vi "Label Targets2.vi"(6 "Edges":cluster{"X":sgl, "Y":sgl}[](array[cluster]), 8 "Line":T1, 9 "Annotate":bool, 10 "Results":T3 {"Score" format="%#_3g"; "Pixels"."Rectangle"."Numeric 5" format="%#_3g"; "Pixels"."Rectangle"."Numeric 3" format="%#_3g"; "Pixels"."Rectangle"."Numeric 2" format="%#_3g"; "Pixels"."Rectangle"."Numeric" format="%#_3g"; "Normalized"."Rectangle"."Numeric 5" format="%#_2g"; "Normalized"."Rectangle"."Numeric 3" format="%#_2g"; "Normalized"."Rectangle"."Numeric 2" format="%#_2g"; "Normalized"."Rectangle"."Numeric" format="%#_2g"; "Normalized"."Center"."?" format="%#_3g"; "Normalized"."Center"."?" format="%#_3g"; "Distance (ft)" format="%#_3g"}, 11 "Image in":T2) -> (3 "Image out":T2)   [LabVIEW 2016]
doc: "Draw text values near or on the particle and draws a square around the target stripes.."
uses:
  <vilib>/vision/Image Controls.llb/IMAQ Image.ctl
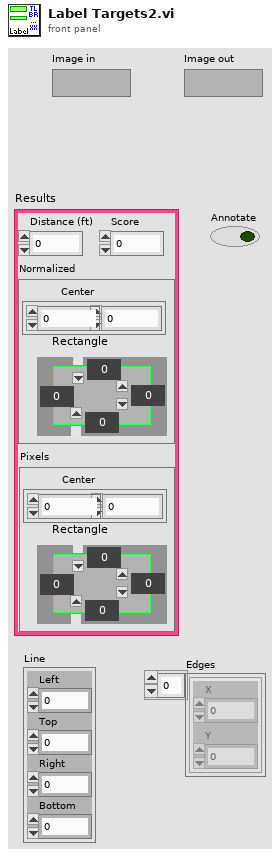
[diagram p1: front panel]
types:
  T1 = cluster{"Left":dbl, "Top":dbl, "Right":dbl, "Bottom":dbl}
  T2 = typedef "IMAQ Image.ctl" = refnum<image>
  T3 = cluster{"Distance (ft)":dbl, "Score":dbl, "Normalized":cluster{"Center":cluster{dbl, dbl}, "Rectangle":cluster{"Numeric":dbl, "Numeric 2":dbl, "Numeric 3":dbl, "Numeric 5":dbl}}, "Pixels":cluster{"Center":cluster{dbl, dbl}, "Rectangle":cluster{"Numeric":dbl, "Numeric 2":dbl, "Numeric 3":dbl, "Numeric 5":dbl}}}
  T4 = cluster{"Desired Font (Application)":enum16{"User-specified Font", "Application Font", "System Font", "Dialog Font"}, "[User-specified Font]":cluster{"Font Name":string, "Size":i16, "Strikeout?":bool, "Italic?":bool, "Underline?":bool, "Outline?":bool, "Shadow?":bool, "Bold?":bool, "Rotation Angle":dbl}, "Horizontal Alignment":i16, "Vertical Alignment":i16}
  T5 = cluster{"Center":cluster{dbl, dbl}, "Rectangle":cluster{"Numeric":dbl, "Numeric 2":dbl, "Numeric 3":dbl, "Numeric 5":dbl}}
  T6 = cluster{"Numeric":dbl, "Numeric 2":dbl, "Numeric 3":dbl, "Numeric 5":dbl}
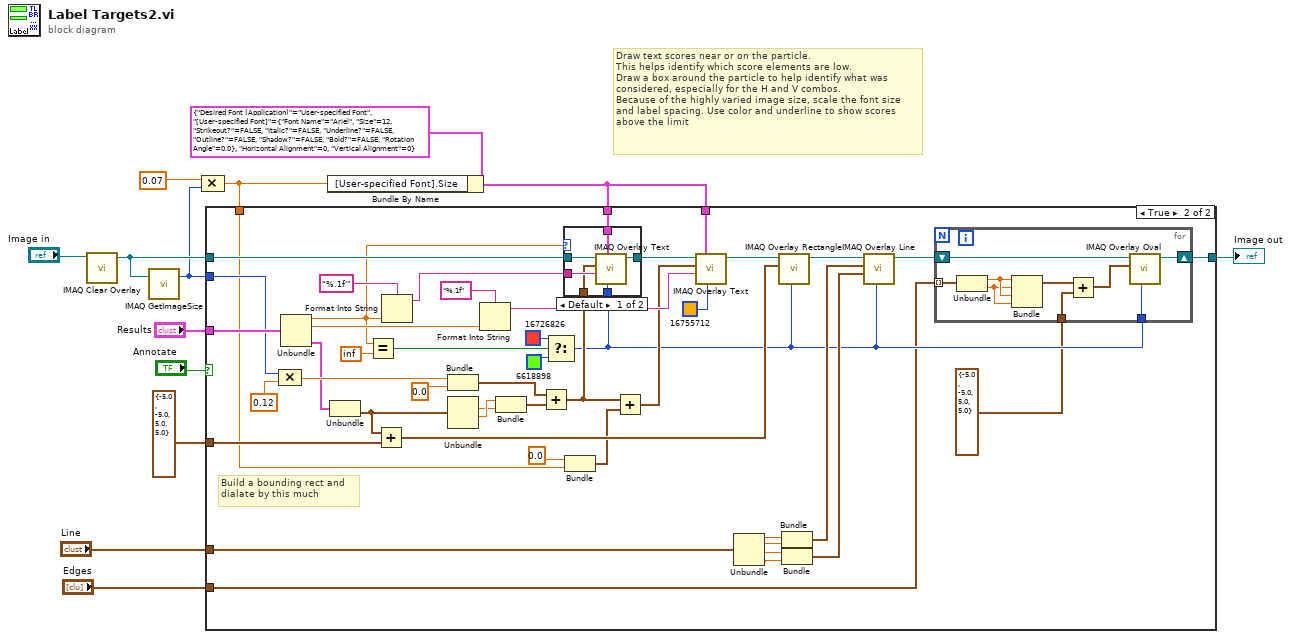
[diagram p0: block diagram]
diagram:
  # "Draw text scores near or on the particle.\nThis helps identify which score elements are low.\nDraw a box around the particle to help identify what was\nconsidered, especially for the H and V combos.\nBecause of the highly varied image size, scale the font size\nand label spacing. Use color and underline to show scores\nabove the limit"
  n1 = call "IMAQ Clear Overlay"("Image"="Image in") -> ("Image Out"=w8:T2)  [unwired: 2 in, 8 out]
  n2 = call "IMAQ GetImageSize"("Image"=w8) -> ("Y Resolution"=w7:i32)  [unwired: 3 in, 2 out]
  n3 = Compound Arithmetic op=MULTIPLY(0.07, w7) -> (w3:dbl)
  n4 = Bundle By Name(cluster=T4 {"Desired Font (Application)"=enum."User-specified Font", "[User-specified Font]"={"Font Name"="Ariel", "Size"=12, "Strikeout?"=FALSE, "Italic?"=FALSE, "Underline?"=FALSE, "Outline?"=FALSE, "Shadow?"=FALSE, "Bold?"=FALSE, "Rotation Angle"=0.0}, "Horizontal Alignment"=0, "Vertical Alignment"=0} ("Font, Size & Style"), "[User-specified Font].Size"=w3) -> (w4:T4)
  n5 = case shown="True" "Annotate" {
    tunnel: [w14 w19] -> w13
    tunnel: "Results" -> [_ w61]
    tunnel: w8 -> [w14 w60]
    tunnel: w4 -> [_ w49]
    tunnel: w7 -> [_ w59]
    tunnel: cluster{dbl, dbl, dbl, dbl} {-5.0, -5.0, 5.0, 5.0} ("output cluster") -> [_ w48]
    tunnel: w4 -> [_ w43]
    tunnel: w3 -> [_ w34]
    tunnel: "Line" -> [_ w28]
    tunnel: "Edges" -> [_ w17]
    frame False {
    }
    frame True {
      # "Build a bounding rect and\ndialate by this much"
      n6 = Compound Arithmetic op=MULTIPLY(w59, 0.12) -> (w52:dbl)
      n7 = Unbundle(w61) -> ("Distance (ft)"=w15:dbl, "Score"=w41:dbl, "Pixels"=w46:T5)  [unwired: 1 out]
      n8 = Unbundle(w46) -> ("Rectangle"=w47:T6)  [unwired: 1 out]
      n9 = Equal?(x=w15, y=inf) -> (x = y?=w30:bool)
      n10 = Add(x=w47, y=w48) -> (x+y=w55:cluster{dbl, dbl, dbl, dbl})
      n11 = Format Into String(format string="%.1f'", w15) -> (resulting string=w50:string)  [unwired: 2 in, 1 out]
      n12 = Bundle(w52, 0.0) -> (w54:cluster{dbl, dbl})  [unwired: 1 in]
      n13 = Unbundle(w47) -> ("Numeric 2"=w57:dbl, "Numeric 3"=w58:dbl)  [unwired: 2 out]
      n14 = Format Into String(format string="%.1f", w41) -> (resulting string=w39:string)  [unwired: 2 in, 1 out]
      n15 = Bundle("Numeric 3"=w58, "Numeric 2"=w57) -> (w56:cluster{"Numeric 3":dbl, "Numeric 2":dbl})  [unwired: 1 in]
      n16 = Add(x=w54, y=w56) -> (x+y=w38:cluster{dbl, dbl})
      n17 = Select(t=u32 16726826 ("Color"), s=w30, f=u32 6618898 ("Color")) -> (s? t:f=w18:u32)
      n18 = case shown="Default" w15 {
        tunnel: w60 -> [w67 w68]
        tunnel: w50 -> [w66 _]
        tunnel: w49 -> [w65 _]
        tunnel: [w64 w68] -> w45
        tunnel: w38 -> [w63 _]
        tunnel: w18 -> [w62 _]
        frame Default {
          n19 = call "IMAQ Overlay Text"("Text Color (black)"=w62, "Font, Size & Style"=w65, "String"=w66, "Origin"=w63, "Image"=w67) -> ("Image Out"=w64:T2)  [unwired: 5 in, 1 out]
        }
        frame 0 {
        }
      }
      n20 = Bundle(0.0, w34) -> (w37:cluster{dbl, dbl})  [unwired: 1 in]
      n21 = Add(x=w38, y=w37) -> (x+y=w35:cluster{dbl, dbl})
      n22 = call "IMAQ Overlay Text"("Text Color (black)"=u32 16755712 ("Color"), "Font, Size & Style"=w43, "String"=w39, "Origin"=w35, "Image"=w45) -> ("Image Out"=w44:T2)  [unwired: 5 in, 1 out]
      n23 = Unbundle(w28) -> ("Left"=w27:dbl, "Top"=w26:dbl, "Right"=w25:dbl, "Bottom"=w24:dbl)
      n24 = call "IMAQ Overlay Rectangle"("Color"=w18, "Rectangle"=w55, "Image"=w44) -> ("Image Out"=w23:T2)  [unwired: 7 in, 1 out]
      n25 = Bundle("Left"=w27, "Top"=w26) -> (w22:cluster{"Left":dbl, "Top":dbl})  [unwired: 1 in]
      n26 = Bundle("Right"=w25, "Bottom"=w24) -> (w21:cluster{"Right":dbl, "Bottom":dbl})  [unwired: 1 in]
      n27 = call "IMAQ Overlay Line"("Color"=w18, "End Point"=w21, "Start Point"=w22, "Image"=w23) -> ("Image Out"=w20:T2)  [unwired: 6 in, 1 out]
      n28 = for {
        shift-right: [w76] -> w19
        shift-left: w20 -> [w77]
        tunnel: w18 -> [w75]
        tunnel: w17 -> [w73] mode=indexing
        tunnel: cluster{"X":sgl, "Y":sgl, "X":sgl, "Y":sgl} {"X"=-5.0, "Y"=-5.0, "X"=5.0, "Y"=5.0} ("output cluster") -> [w69]
        n29 = Unbundle(w73) -> ("X"=w72:sgl, "Y"=w71:sgl)
        n30 = Bundle("X"=w72, "Y"=w71, "X"=w72, "Y"=w71) -> (w70:cluster{"X":sgl, "Y":sgl, "X":sgl, "Y":sgl})  [unwired: 1 in]
        n31 = Add(x=w70, y=w69) -> (x+y=w74:cluster{"X":sgl, "Y":sgl, "X":sgl, "Y":sgl})
        n32 = call "IMAQ Overlay Oval"("Color"=w75, "Bounding Rectangle"=w74, "Image"=w77) -> ("Image Out"=w76:T2)  [unwired: 7 in, 1 out]
      }
    }
  }
  "Image out" <- w13
